vi "DO Coils Group UI.vi"(8 "error in (no error)":errorcluster, 11 "Node Ptr":T2 format="%.0x") -> (0 "error out":errorcluster)   [LabVIEW 2015, in "Modbus Master System Explorer.lvlib"]
uses:
  Modbus Master System Explorer.lvlib
  <vilib>/NI Veristand/Custom Device API/Custom Device Item Ref.ctl
  SubVIs/Conflict Table.ctl
  <vilib>/NI VeriStand/Custom Device API/Custom Device API.lvlib
  <vilib>/NI VeriStand/Custom Device Tools/Custom Device Utility Library/Custom Device Utility Library.lvlib
panel:
  in  "Delete Multiple":bool
  in  "Bulk Add Coils":bool
  in  "Add Coil":bool
  out "Conflicting Coil Mappings":T1
  in  "Header":cluster{"Section Name":string}={"Section Name"="Coil Group Settings"}
  in  "Description":string
  in  "Name":string
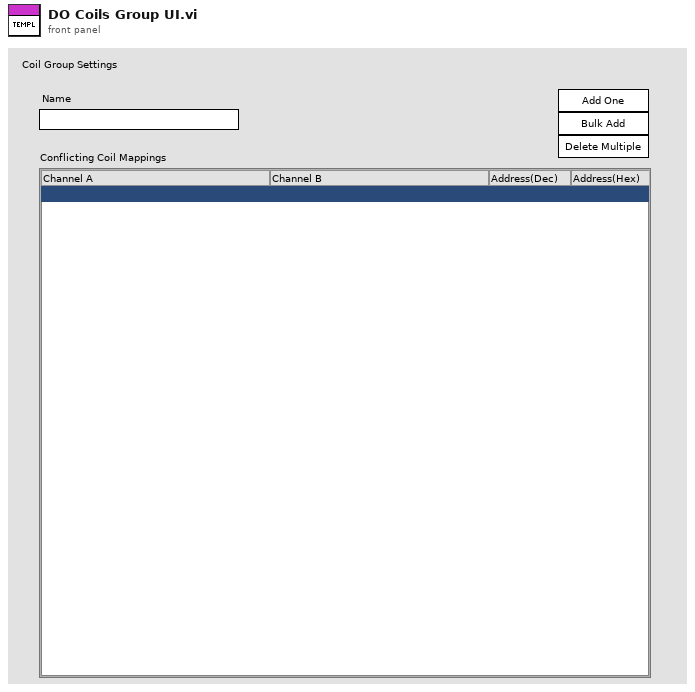
[diagram p1: front panel]
types:
  T1 = typedef "Modbus Master System Explorer.lvlib/Conflict Table.ctl" = i32
  T2 = typedef "Custom Device API.lvlib/Custom Device Item Ref.ctl" = u64
  T3 = typedef "Custom Device API.lvlib/Custom Device Item Info.ctl" = cluster{"Name":string, "Is Channel":bool, "GUID":string, "Is Waveform":bool}
  T4 = cluster{"Name":string, "Name":string, "Mapping":u16}[]
  T5 = typedef "Custom Device API.lvlib/Custom Device Commands.ctl" = enum16{"Default", "Item renamed", "Shutdown", "Dynamic button pressed"}
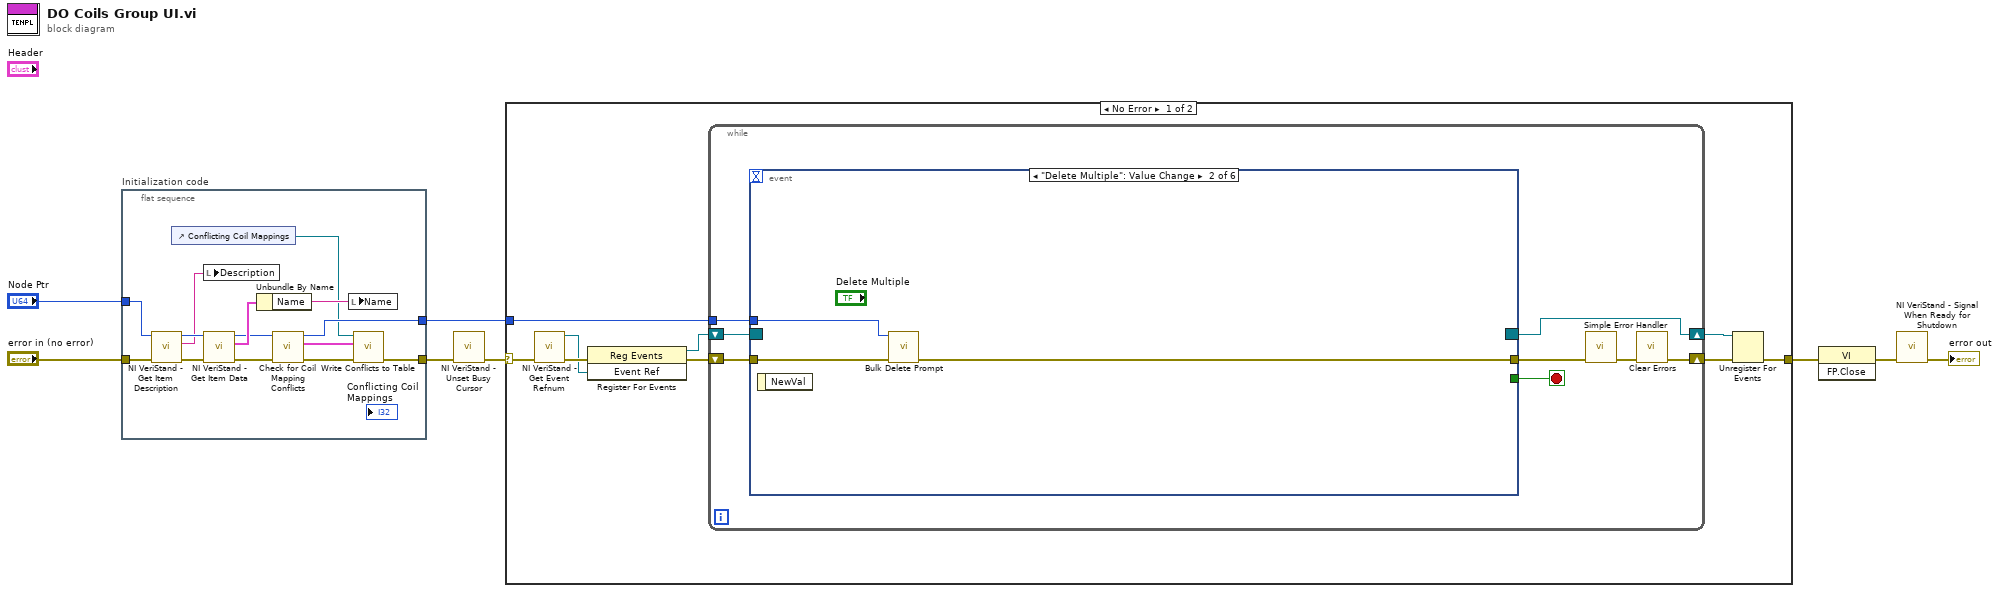
[diagram p0: block diagram]
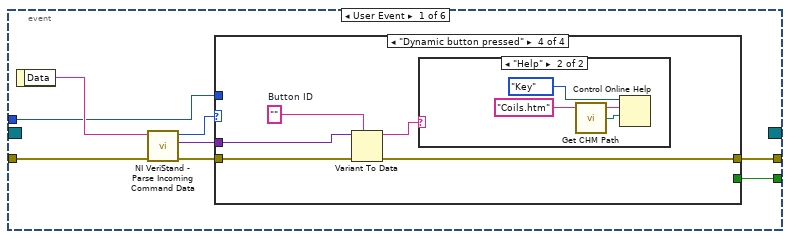
[diagram p2: hidden frame]
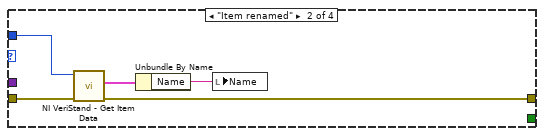
[diagram p4: hidden frame]
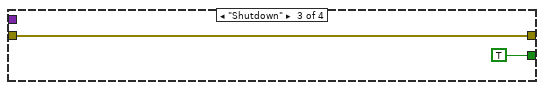
[diagram p5: hidden frame]
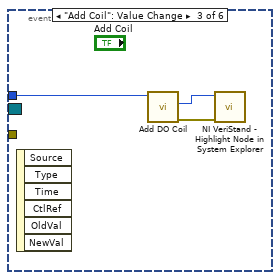
[diagram p7: hidden frame]
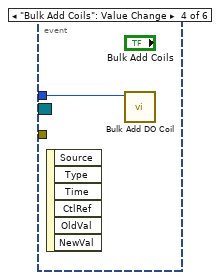
[diagram p8: hidden frame]
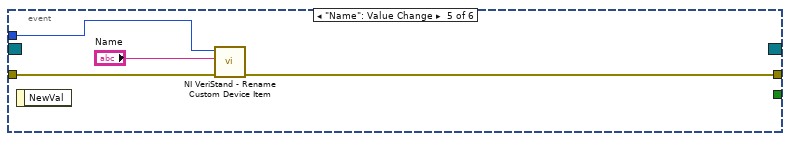
[diagram p9: hidden frame]
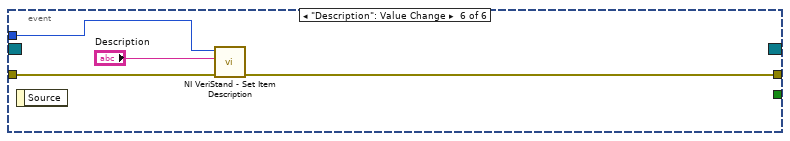
[diagram p10: hidden frame]
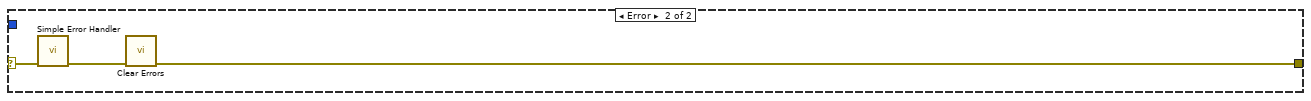
[diagram p11: hidden frame]
diagram:
  n1 = flat-sequence "Initialization code" {
    tunnel: "error in (no error)" -> [w21]
    tunnel: "Node Ptr" -> [w20]
    tunnel: [w9] -> w4
    tunnel: [w13] -> w1
    frame #0 {
      n2 = call <vilib>:"NI VeriStand - Get Item Description.vi"("error in (no error)"=w21, "Item Ref in"=w20) -> ("error out"=w18:errorcluster, "Description"=w19:string, "Item Ref out"=w22:T2)  [unwired: 7 out]
      n3 = control-ref of="Conflicting Coil Mappings"() -> (w12:refnum<vi>)
      n4 = local write "Description"(w19) -> ()
      n5 = call <vilib>:"NI VeriStand - Get Item Data.vi"("error in (no error)"=w18, "Item Ref in"=w22) -> ("error out"=w14:errorcluster, "Item Info"=w17:T3, "Item Ref out"=w15:T2)  [unwired: 7 out]
      n6 = Unbundle By Name(w17) -> ("Name"=w16:string)
      n7 = call "Check for Coil Mapping Conflicts.vi"("error in (no error)"=w14, "Coiil Group Ref in"=w15) -> ("error out"=w10:errorcluster, "Conflicts"=w11:T4, "Coil Group Ref out"=w13:T2)  [unwired: 6 in, 1 out]
      n8 = local write "Name"(w16) -> ()
      n9 = call "Write Conflicts to Table.vi"("error in (no error)"=w10, "Conflicts"=w11, "MC Listbox Ref"=w12) -> ("error out"=w9:errorcluster)  [unwired: 8 in]
    }
  }
  n10 = call <vilib>:"NI VeriStand - Unset Busy Cursor.vi"("error in (no error)"=w4) -> ("error out"=w3:errorcluster)  [unwired: 10 out]
  n11 = case shown="No Error" w3 {
    selector: w3 -> [w23 w81]
    tunnel: [w28 w79] -> w8
    tunnel: w1 -> [w24 _]
    frame No Error {
      n12 = call <vilib>:"NI VeriStand - Get Event Refnum.vi"("error in (no error)"=w23) -> ("error out"=w31:errorcluster, "Event Ref"=w27:refnum<user-event>)  [unwired: 9 out]
      n13 = register-events(error in=w31, w27) -> (reference out=w25:refnum<event-registration>, error out=w26:errorcluster)  [unwired: 1 in]
      n14 = while {
        tunnel: w24 -> [w35]
        shift-right: [w32] -> w29
        shift-left: w26 -> [w38]
        shift-right: [w39] -> w30
        shift-left: w25 -> [w37]
        stop <- w36 stop-if-true
        n15 = event shown="[1] \"Delete Multiple\": Value Change" {
          selector: w37 -> [_ _ _ _ _ _]
          dyn-events: [_ _ _ _ _ _] -> w39
          timeout: _ -> [_ _ _ _ _ _]
          tunnel: w38 -> [w47 w65 _ _ w74 w77]
          tunnel: [w43 _ _ _ _ _] -> w36
          tunnel: [w42 w64 _ _ w73 w76] -> w34
          tunnel: w35 -> [w41 w66 w67 w70 w72 w78]
          event User Event {
            n16 = event-data() -> ("Data"=w46:string)  [unwired: 1 out]
            n17 = call <vilib>:"NI VeriStand - Parse Incoming Command Data.vi"("error in (no error)"=w47, "Incoming data"=w46) -> ("error out"=w45:errorcluster, "Outgoing data"=w40:variant, "Action"=w44:T5)  [unwired: 7 out]
            n18 = case shown="\"Dynamic button pressed\"" w44 {
              tunnel: w45 -> [w48 w53 w54 w60]
              tunnel: [_ _ TRUE _] -> w43
              tunnel: [w48 w50 w54 w57] -> w42
              tunnel: w41 -> [_ w52 _ _]
              tunnel: w40 -> [_ _ _ w59]
              frame "Default", Default {
              }
              frame "Item renamed" {
                n19 = call <vilib>:"NI VeriStand - Get Item Data.vi"("error in (no error)"=w53, "Item Ref in"=w52) -> ("error out"=w50:errorcluster, "Item Info"=w51:T3)  [unwired: 8 out]
                n20 = Unbundle By Name(w51) -> ("Name"=w49:string)
                n21 = local write "Name"(w49) -> ()
              }
              frame "Shutdown" {
              }
              frame "Dynamic button pressed" {
                w58 = ""  # Button ID
                n22 = Variant To Data(error in=w60, type=w58, Variant=w59) -> (data=w56:string, error out=w57:errorcluster)
                n23 = case shown="\"Help\"" w56 {
                  frame Default {
                  }
                  frame "Help" {
                    n24 = call "Get CHM Path.vi"() -> ("appended path"=w63:path)
                    n25 = Control Online Help(2:w63, 3:"Coils.htm" ("String to search for"), 4:enum16{"Contents", "Key", "Close"}."Key" ("Operation")) -> ()  [unwired: 1 in, 1 out]
                  }
                }
              }
            }
          }
          event "Delete Multiple": Value Change {
            n26 = event-data() -> ()  [unwired: 2 out]
            n27 = call "Bulk Delete Prompt.vi"("error in (no error)"=w65, "Item Ref in"=w66) -> ("error out"=w64:errorcluster)  [unwired: 9 in]
          }
          event "Add Coil": Value Change {
            n28 = event-data() -> ()  [unwired: 7 out]
            n29 = call "Add DO Coil.vi"("Node Ref In"=w67) -> ("error out"=w68:errorcluster, "Channel Ref"=w69:T2)  [unwired: 8 in, 1 out]
            n30 = call <vilib>:"NI VeriStand - Highlight Node in System Explorer.vi"("error in (no error)"=w68, "Item Ref in"=w69) -> ()  [unwired: 8 in, 2 out]
          }
          event "Bulk Add Coils": Value Change {
            n31 = event-data() -> ()  [unwired: 7 out]
            n32 = call "Bulk Add DO Coil.vi"("Node Ptr"=w70) -> ()  [unwired: 11 in]
          }
          event "Name": Value Change {
            n33 = event-data() -> ()  [unwired: 2 out]
            n34 = call <vilib>:"NI VeriStand - Rename Custom Device Item.vi"("error in (no error)"=w74, "New Name"="Name", "Item Ref in"=w72) -> ("error out"=w73:errorcluster)  [unwired: 1 in, 7 out]
          }
          event "Description": Value Change {
            n35 = event-data() -> ()  [unwired: 2 out]
            n36 = call <vilib>:"NI VeriStand - Set Item Description.vi"("error in (no error)"=w77, "Description"="Description", "Item Ref in"=w78) -> ("error out"=w76:errorcluster)  [unwired: 8 out]
          }
        }
        n37 = call <vilib>:"Simple Error Handler.vi"("error in (no error)"=w34) -> ("error out"=w33:errorcluster)  [unwired: 1 in, 7 out]
        n38 = call <vilib>:"Clear Errors.vi"("error in (no error)"=w33) -> ("error out"=w32:errorcluster)  [unwired: 1 in, 5 out]
      }
      n39 = Unregister For Events(event registration refnum=w30, error in=w29) -> (error out=w28:errorcluster)
    }
    frame Error {
      n40 = call <vilib>:"Simple Error Handler.vi"("error in (no error)"=w81) -> ("error out"=w80:errorcluster)  [unwired: 1 in, 7 out]
      n41 = call <vilib>:"Clear Errors.vi"("error in (no error)"=w80) -> ("error out"=w79:errorcluster)  [unwired: 1 in, 5 out]
    }
  }
  n42 = invoke class="VI" method="FP.Close"(error in=w8) -> (error out=w7:errorcluster)  [unwired: 2 in, 2 out]
  n43 = call <vilib>:"NI VeriStand - Signal When Ready for Shutdown.vi"("error in (no error)"=w7) -> ("error out"=→"error out":errorcluster)  [unwired: 10 out]
